vi "Do Event Report.vi"(8 "error in (no error)":errorcluster, 9 "Event Data":variant, 10 "Scope Events":T1, 11 "Caller Enqueuer":refnum<class "Message Enqueuer.lvclass">) -> (0 "error out":errorcluster, 3 "Message Enqueuer out":refnum<class "Message Enqueuer.lvclass">)   [LabVIEW 2020, in "Actor_Scope.lvlib" / "Actor_Scope.lvclass"]
uses:
  Actor_Scope.lvclass
  <vilib>/ActorFramework/Message Enqueuer/Message Enqueuer.lvclass
  Scope_Event.ctl
  I_Scope Messages/Scope Report Event Msg/Scope Report Event Msg.lvclass/Scope Report Event Msg.ctl
  <vilib>/ActorFramework/Message Enqueuer/Message Enqueuer.lvclass/Message Enqueuer.ctl
  <vilib>/ActorFramework/Message Enqueuer/Enqueue.vi
  I_Scope Messages/Scope Report Event Msg/Scope Report Event Msg.lvclass
  C:/Program Files/National Instruments/LabVIEW 2020/vi.lib/ActorFramework/Message/Message.lvclass
  <vilib>/ActorFramework/Message Priority Queue/Priority Enqueue.vi
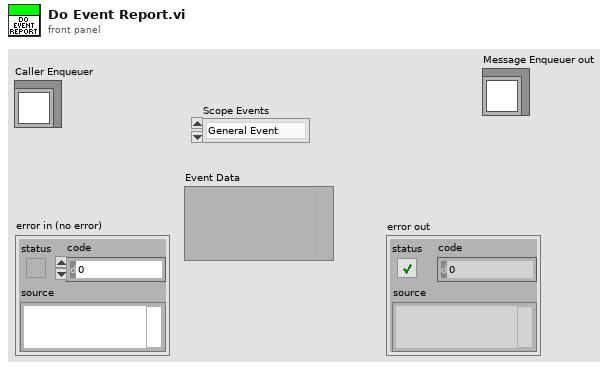
[diagram p1: front panel]
types:
  T1 = typedef "Actor_Scope.lvlib/Actor_Scope.lvclass/Scope_Event.ctl" = enum16{"General Event", "Inited", "Error", "Res Read complete", "Wfm Acq Complete"}
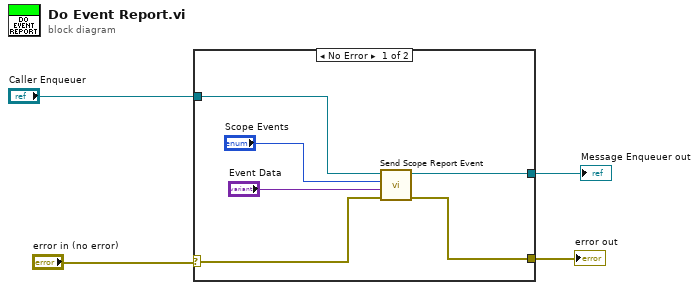
[diagram p0: block diagram]
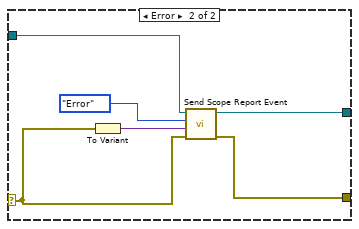
[diagram p2: hidden frame]
diagram:
  n1 = case shown="No Error" "error in (no error)" {
    selector: "error in (no error)" -> [w7 w12]
    tunnel: "Caller Enqueuer" -> [w9 w14]
    tunnel: [w6 w11] -> w2
    tunnel: [w5 w13] -> w1
    frame No Error {
      n2 = call "Send Scope Report Event.vi"("error in (no error)"=w7, "Event Data"="Event Data", "Scope Events"="Scope Events", "Message Enqueuer"=w9) -> ("error out"=w6:errorcluster, "Message Enqueuer out"=w5:refnum<class "Message Enqueuer.lvclass">)  [unwired: 6 in]
    }
    frame Error {
      n3 = To Variant(anything=w12) -> (Variant=w16:variant)
      n4 = call "Send Scope Report Event.vi"("error in (no error)"=w12, "Event Data"=w16, "Scope Events"=Scope_Event."Error", "Message Enqueuer"=w14) -> ("error out"=w11:errorcluster, "Message Enqueuer out"=w13:refnum<class "Message Enqueuer.lvclass">)  [unwired: 6 in]
    }
  }
  "error out" <- w2
  "Message Enqueuer out" <- w1
